vi "main.vi"() -> ()   [LabVIEW 2012]
uses:
  src/_gStop.vi
  src/GlobalStop(dev).lvlib
panel:
  in  "gen error":bool
  out "error out":errorcluster
  out "loop4":i32
  in  "stop 2":bool
  out "loop3":i32
  out "loop2":i32
  out "loop1":i32
  in  "stop":bool
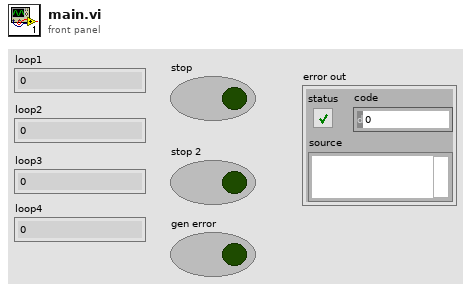
[diagram p1: front panel]
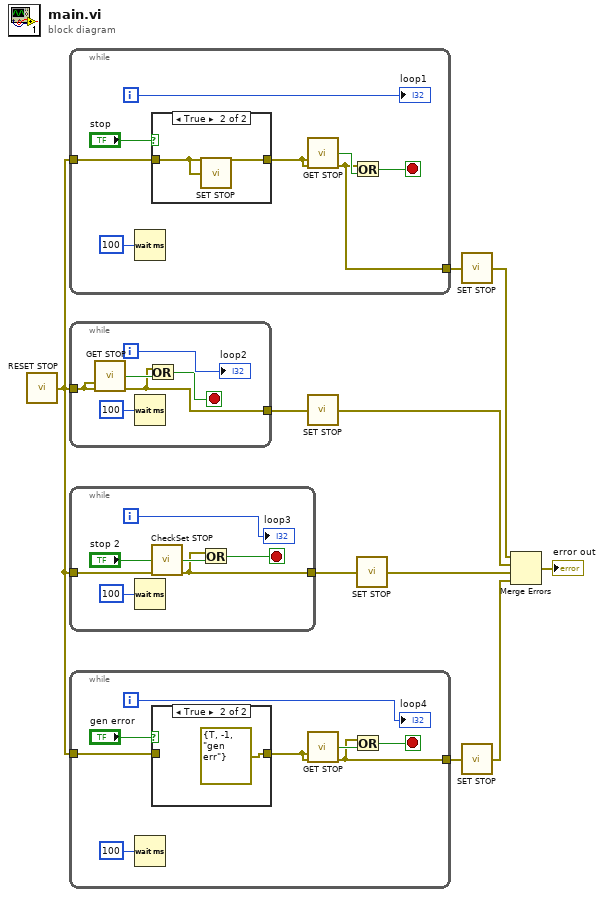
[diagram p0: block diagram]
diagram:
  n1 = call "RESET STOP.vi"() -> ("error out"=w3:errorcluster)  [unwired: 5 in]
  n2 = while {
    tunnel: w3 -> [w17]
    tunnel: [w11] -> w10
    i -> [w15]
    stop <- w12 stop-if-true
    n3 = Wait (ms)(milliseconds to wait=100) -> ()  [unwired: 1 out]
    n4 = case shown="True" "stop" {
      tunnel: w17 -> [w18 w19]
      tunnel: [w18 w19] -> w11
      frame False {
      }
      frame True {
        n5 = call "SET STOP.vi"("error in (no error)"=w19) -> ()  [unwired: 4 in, 1 out]
      }
    }
    n6 = call "GET STOP.vi"("error in (no error)"=w11) -> ("Boolean"=w13:bool)  [unwired: 13 in, 1 out]
    n7 = Or(x=w11, y=w13) -> (x .or. y?=w12:bool)
    "loop1" <- w15
  }
  n8 = while {
    tunnel: w3 -> [w20]
    tunnel: [w20] -> w8
    i -> [w24]
    stop <- w21 stop-if-true
    n9 = call "GET STOP.vi"("error in (no error)"=w20) -> ("Boolean"=w22:bool)  [unwired: 13 in, 1 out]
    n10 = Wait (ms)(milliseconds to wait=100) -> ()  [unwired: 1 out]
    n11 = Or(x=w20, y=w22) -> (x .or. y?=w21:bool)
    "loop2" <- w24
  }
  n12 = while {
    tunnel: w3 -> [w25]
    tunnel: [w25] -> w6
    i -> [w30]
    stop <- w26 stop-if-true
    n13 = Wait (ms)(milliseconds to wait=100) -> ()  [unwired: 1 out]
    n14 = call "CheckSet STOP.vi"("stop value"="stop 2") -> ("Boolean"=w27:bool)  [unwired: 13 in, 1 out]
    n15 = Or(x=w25, y=w27) -> (x .or. y?=w26:bool)
    "loop3" <- w30
  }
  n16 = while {
    tunnel: w3 -> [w34]
    tunnel: [w31] -> w4
    i -> [w37]
    stop <- w32 stop-if-true
    n17 = Wait (ms)(milliseconds to wait=100) -> ()  [unwired: 1 out]
    n18 = case shown="True" "gen error" {
      tunnel: w34 -> [w38 _]
      tunnel: [w38 errorcluster {"status"=TRUE, "code"=-1, "source"="gen err"} ("error out")] -> w31
      frame False {
      }
      frame True {
      }
    }
    n19 = call "GET STOP.vi"("error in (no error)"=w31) -> ("Boolean"=w33:bool)  [unwired: 13 in, 1 out]
    n20 = Or(x=w31, y=w33) -> (x .or. y?=w32:bool)
    "loop4" <- w37
  }
  n21 = call "SET STOP.vi"("error in (no error)"=w8) -> ("error out"=w7:errorcluster)  [unwired: 4 in]
  n22 = call "SET STOP.vi"("error in (no error)"=w6) -> ("error out"=w5:errorcluster)  [unwired: 4 in]
  n23 = call "SET STOP.vi"("error in (no error)"=w10) -> ("error out"=w9:errorcluster)  [unwired: 4 in]
  n24 = call "SET STOP.vi"("error in (no error)"=w4) -> ("error out"=w2:errorcluster)  [unwired: 4 in]
  n25 = Merge Errors(w9, w7, w5, w2) -> (→"error out":errorcluster)
